vi "RESTful Validate Class Type.vi"(8 "error in (no error)":errorcluster, 9 "Service VI Type":T1, 10 "indicator?":bool, 11 "Variant":variant) -> (0 "error out":errorcluster, 2 "valid?":bool, 3 "ignore terminal?":bool)   [LabVIEW 2020]
uses:
  <vilib>/AppBuilder/AB_Classes/Source/RESTfulVI/Configure_RESTfulVI/AB_RESTful_VIType.ctl
  <vilib>/Utility/VariantDataType/VariantType.lvlib
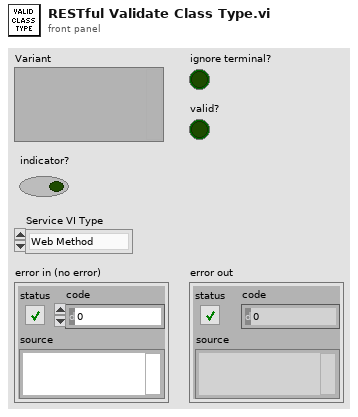
[diagram p1: front panel]
types:
  T1 = typedef "AB_RESTful_VIType.ctl" = enum32{"Web Method", "Auxiliary", "eng_Internal", "eng_Content"}
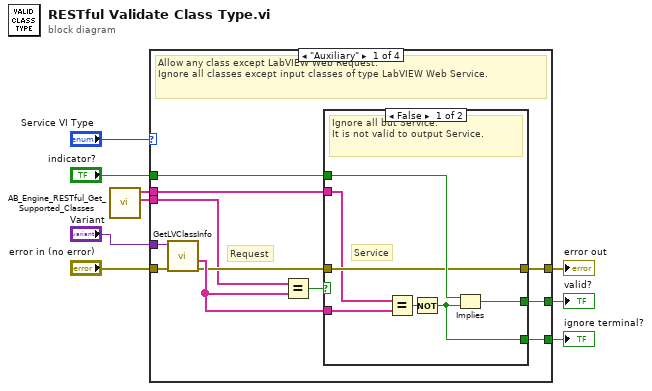
[diagram p0: block diagram]
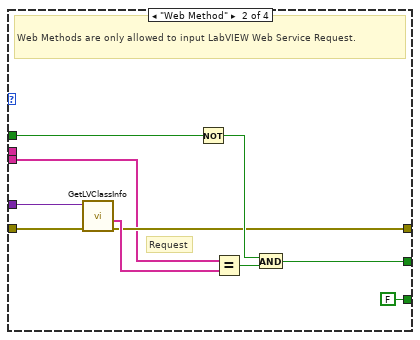
[diagram p3: hidden frame]
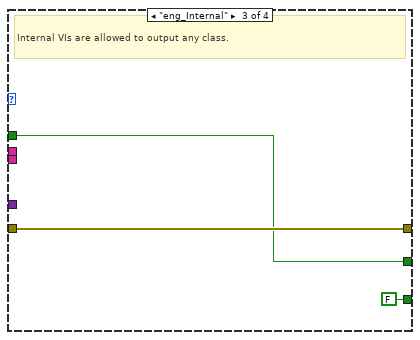
[diagram p4: hidden frame]
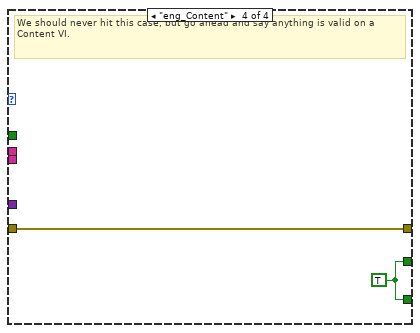
[diagram p5: hidden frame]
diagram:
  n1 = call <vilib>:"AB_Engine_RESTful_Get_Supported_Classes.vi"() -> ("Web Request"=w1:string[], "Web Service"=w2:string[])  [unwired: 10 in]
  n2 = case shown="\"Auxiliary\"" "Service VI Type" {
    tunnel: "indicator?" -> [w13 w33 w41 _]
    tunnel: "Variant" -> [w19 w38 _ _]
    tunnel: "error in (no error)" -> [w20 w39 w42 w44]
    tunnel: [w17 w34 w41 w43] -> w4
    tunnel: [w16 FALSE FALSE w43] -> w3
    tunnel: [w15 w31 w42 w44] -> w8
    tunnel: w2 -> [w10 _ _ _]
    tunnel: w1 -> [w11 w30 _ _]
    frame "Auxiliary" {
      # "Request"
      # "Allow any class except LabVIEW Web Request.\nIgnore all classes except input classes of type LabVIEW Web Service."
      n3 = call <vilib>:"GetLVClassInfo.vi"("error in (no error)"=w20, "Variant"=w19) -> ("error out"=w12:errorcluster, "Fully Qualified LV Class Name"=w14:string[])  [unwired: 7 in, 1 out]
      n4 = Equal?(x=w11, y=w14) -> (x = y?=w18:bool)
      n5 = case shown="False" w18 {
        tunnel: [w23 w29] -> w17
        tunnel: [w24 w29] -> w16
        tunnel: w12 -> [w22 w28]
        tunnel: [w22 w28] -> w15
        tunnel: w14 -> [w27 _]
        tunnel: w13 -> [w25 _]
        tunnel: w10 -> [w21 _]
        frame False {
          # "Service"
          # "Ignore all but Service.\nIt is not valid to output Service."
          n6 = Equal?(x=w21, y=w27) -> (x = y?=w26:bool)
          n7 = Not(x=w26) -> (.not. x?=w24:bool)
          n8 = Implies(1:w24, 2:w25) -> (0:w23:bool)
        }
        frame True {
          w29 = FALSE
          # "Request class is not allowed."
        }
      }
    }
    frame "Web Method" {
      # "Request"
      # "Web Methods are only allowed to input LabVIEW Web Service Request."
      n9 = call <vilib>:"GetLVClassInfo.vi"("error in (no error)"=w39, "Variant"=w38) -> ("error out"=w31:errorcluster, "Fully Qualified LV Class Name"=w37:string[])  [unwired: 7 in, 1 out]
      n10 = Not(x=w33) -> (.not. x?=w32:bool)
      n11 = Equal?(x=w30, y=w37) -> (x = y?=w36:bool)
      n12 = And(x=w32, y=w36) -> (x .and. y?=w34:bool)
    }
    frame "eng_Internal" {
      # "Internal VIs are allowed to output any class."
    }
    frame "eng_Content" {
      w43 = TRUE ("indicator?")
      # "We should never hit this case, but go ahead and say anything is valid on a Content VI."
    }
  }
  "error out" <- w8
  "valid?" <- w4
  "ignore terminal?" <- w3
